vi "Get Name.vi"(8 "error in (no error)":errorcluster, 11 "CIPC Reference":u64) -> (0 "error out":errorcluster, 3 "Name":string)   [LabVIEW 2021, in "CIF_NI_CIPC.lvlib"]
uses:
  CIF_NI_CIPC.lvlib
  <vilib>/Utility/error.llb/Trim Whitespace.vi
  <vilib>/Utility/error.llb/Error Cluster From Error Code.vi
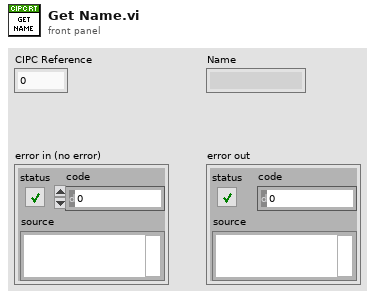
[diagram p1: front panel]
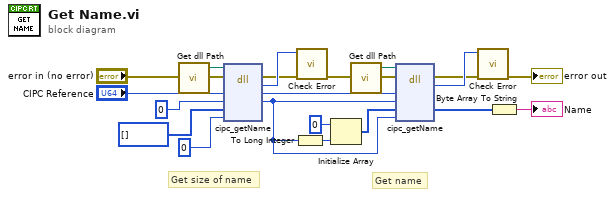
[diagram p0: block diagram]
diagram:
  # "Get name"
  # "Get size of name"
  n1 = call "Get dll Path.vi"() -> ("appended path"=w4:path)  [unwired: 5 in]
  n2 = dll-call lib="libnicipc.*" fn="cipc_getName"(path in=w4, error in="error in (no error)", "cipc_buffer_ref"="CIPC Reference", "name_size"=u32 0 ("descr_size"), "el_name"=u8[] [] ("initialized array"), "el_name_maxsize"=u32 0 ("el_descr_maxsize")) -> (error out=w19:errorcluster, "return type"=w20:i32, "cipc_buffer_ref"=w15:u64, "name_size"=w2:u32)  [unwired: 3 in, 1 out]
  n3 = To Long Integer(number=w2) -> (32bit integer=w5:i32)
  n4 = call "Check Error.vi"("error in (no error)"=w19, "Error Code"=w20) -> ("error out"=w16:errorcluster)  [unwired: 9 in]
  n5 = Initialize Array(u8 0, w5) -> (w10:u8[])
  n6 = call "Get dll Path.vi"() -> ("appended path"=w3:path)  [unwired: 5 in]
  n7 = dll-call lib="libnicipc.*" fn="cipc_getName"(path in=w3, error in=w16, "cipc_buffer_ref"=w15, "name_size"=w2, "el_name"=w10, "el_name_maxsize"=w2) -> (error out=w17:errorcluster, "return type"=w18:i32, "el_name"=w1:u8[])  [unwired: 4 in, 1 out]
  n8 = call "Check Error.vi"("error in (no error)"=w17, "Error Code"=w18) -> ("error out"=→"error out":errorcluster)  [unwired: 9 in]
  n9 = Byte Array To String(unsigned byte array=w1) -> (string=→"Name":string)
